vi "Read Frame.vi"(8 "error in (no error)":errorcluster, 9 "timeout (1000 ms)":i32=1000, 11 "Connection.WS":refnum<class "Connection.WS.lvclass">) -> (0 "error out":errorcluster, 1 "timed out":bool, 2 "Bytes":u8[](array[numeric]) format="%08b", 3 "Connection.WS":refnum<class "Connection.WS.lvclass">, 4 "connected":bool, 5 "Frame Type":T1=2 items=["continuation"=0, "text"=1, "binary"=2, "close"=8, "ping"=9, "pong"=10])   [LabVIEW 2013, in "Connection.WS_GOSPL.lvlib" / "Connection.WS.lvclass"]
uses:
  Connection.WS.lvclass
  Websocket Frame Type -- ring.ctl
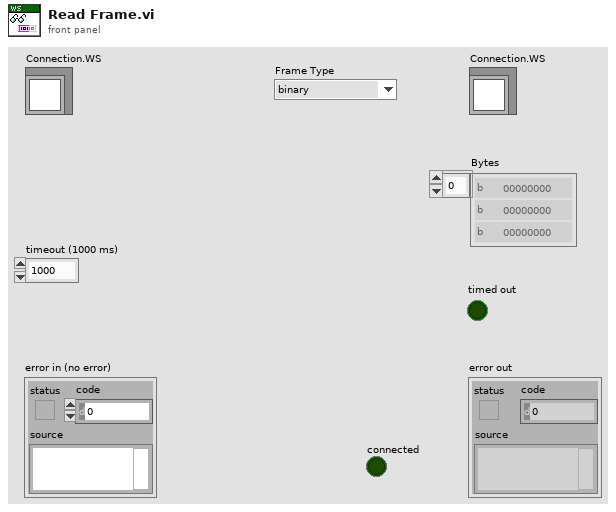
[diagram p1: front panel]
types:
  T1 = typedef "Connection.WS_GOSPL.lvlib/Connection.WS.lvclass/Websocket Frame Type -- ring.ctl" = u8
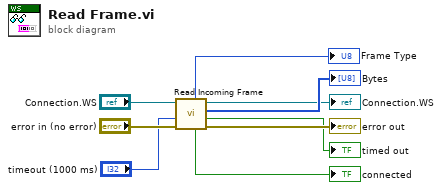
[diagram p0: block diagram]
diagram:
  n1 = call "Read Incoming Frame.vi"("error in (no error)"="error in (no error)", "timeout (1000 ms)"="timeout (1000 ms)", "Connection.TCP"="Connection.WS") -> ("error out"=→"error out":errorcluster, "timed out"=→"timed out":bool, "Bytes"=→"Bytes":u8[], "Connection.TCP"=→"Connection.WS":refnum<class "Connection.WS.lvclass">, "connected"=→"connected":bool, "Frame type"=→"Frame Type":T1)  [unwired: 3 in]
